vi "data length.vi"() -> ()   [LabVIEW 2013]
panel:
  in  "data length":i32[](array[numeric])
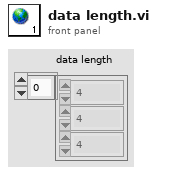
[diagram p1: front panel]
diagram:
